vi "ProgressWindowDialog.vi"(0 "LibWriter":refnum<class "LibWriter.lvclass">, 5 "error in (no error)":errorcluster) -> (19 "error out":errorcluster)   [LabVIEW 2014, in "LibWriter.lvclass"]
uses:
  <resource>/Framework/Providers/Open_GDS/ClassProviders/LibProvider_BaseClassInterface/LibWriter_class/ClassWriter_class/LibWriter.lvclass
  <vilib>/picture/picture.llb/imagedata.ctl
  <resource>/Framework/Providers/Open_GDS/ClassProviders/LibProvider_BaseClassInterface/LibWriter_class/ClassWriter_class/LibWriter.lvclass/LibWriter.ctl
panel:
  out "Message":string
  out "Bar":picture
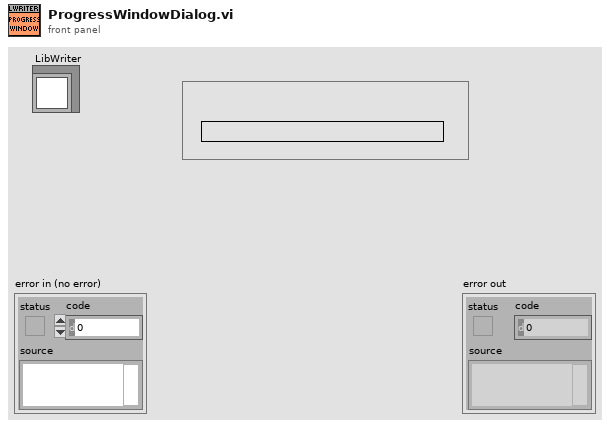
[diagram p1: front panel]
types:
  T1 = typedef "imagedata.ctl" = cluster{"image type":i32, "image depth":i32, "image":u8[], "mask":u8[], "colors":u32[], "Rectangle":cluster{"left":i16, "top":i16, "right":i16, "bottom":i16}}
  T2 = cluster{"i":i32, "end":i32, "Right":bool, "Event":refnum<event-registration>}
  T3 = enum32{"Invalid", "Default", "Floating", "Floating/Auto-Hide", "Modal"}
  T4 = cluster{"left":i16, "top":i16, "right":i16, "bottom":i16}
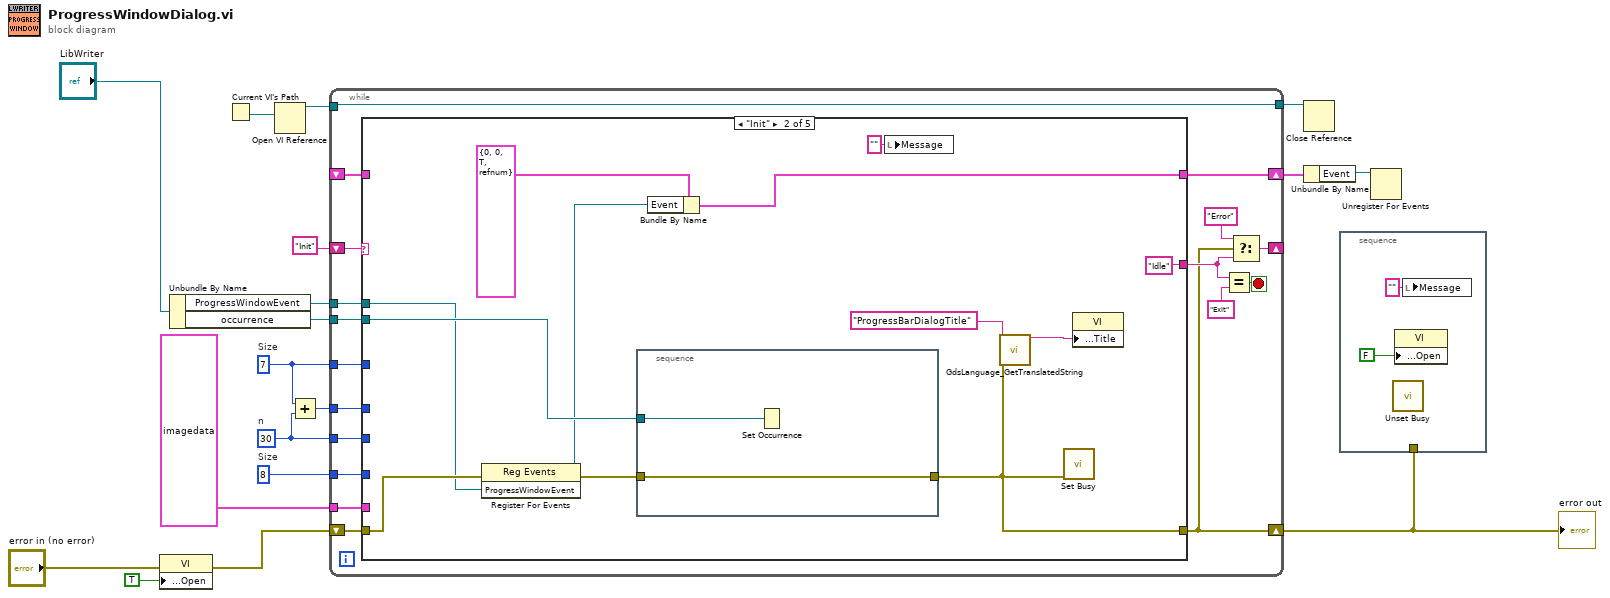
[diagram p0: block diagram]
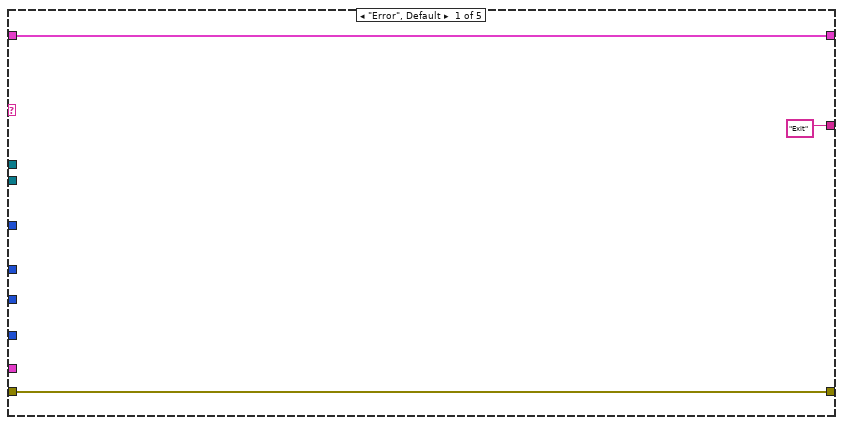
[diagram p2: hidden frame]
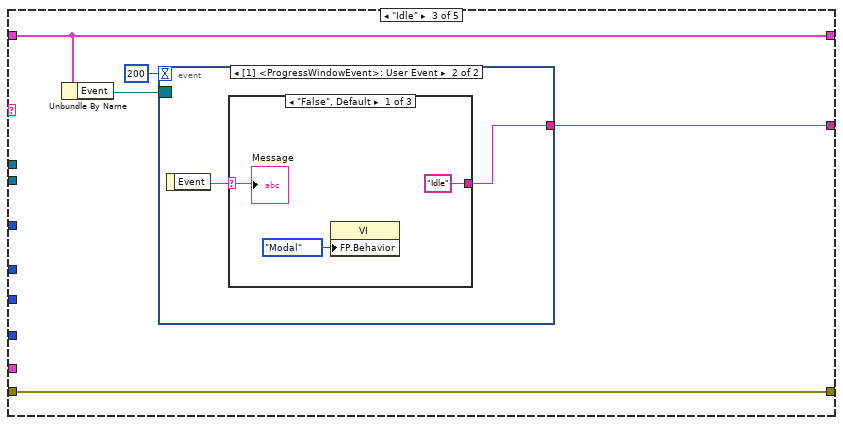
[diagram p3: hidden frame]
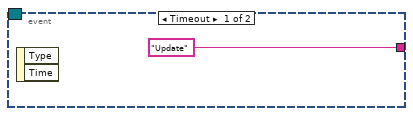
[diagram p4: hidden frame]
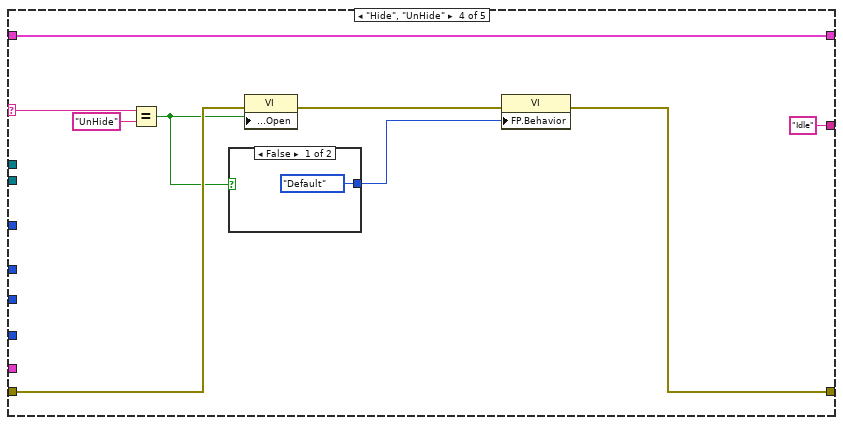
[diagram p7: hidden frame]
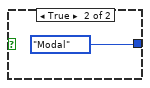
[diagram p8: hidden frame]
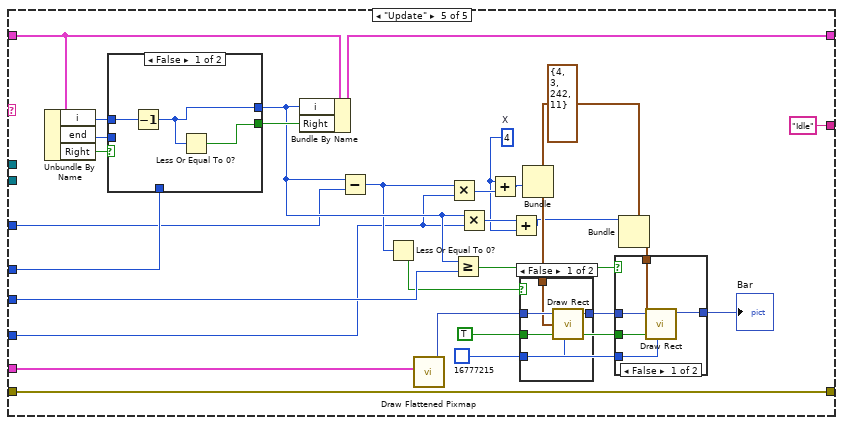
[diagram p9: hidden frame]
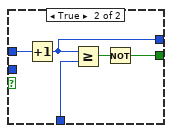
[diagram p12: hidden frame]
diagram:
  w11 = 7  # Size
  w12 = 8  # Size
  w10 = 30  # n
  n1 = property class="VI"(error in="error in (no error)", "Front Panel.Open"=TRUE ("Front Panel Window:Open")) -> (error out=w6:errorcluster)  [unwired: 1 in, 1 out]
  n2 = Unbundle By Name("LibWriter") -> ("ProgressWindowEvent"=w16:refnum<user-event>, "occurrence"=w13:refnum<k4>)
  n3 = Current VI's Path() -> (path=w2:path)
  n4 = Open VI Reference(vi path=w2) -> (vi reference=w3:refnum<vi>)  [unwired: 5 in, 1 out]
  n5 = Add(x=w11, y=w10) -> (x+y=w9:i32)
  n6 = while {
    shift-right: [w29] -> w7
    shift-left: w6 -> [w36]
    shift-right: [w34] -> _
    shift-left: "Init" -> [w35]
    shift-right: [w28] -> w15
    shift-left: _ -> [w27]
    tunnel: w16 -> [w26]
    tunnel: w13 -> [w25]
    tunnel: w12 -> [w24]
    tunnel: w10 -> [w23]
    tunnel: w11 -> [w22]
    tunnel: T1 {"image type"=0, "image depth"=24, "image"=array[9555 elements], "mask"=[], "colors"=[], "Rectangle"={"left"=0, "top"=0, "right"=245, "bottom"=13}} ("image data") -> [w21]
    tunnel: w9 -> [w20]
    tunnel: w3 -> [w19]
    tunnel: [w19] -> w1
    stop <- w33 stop-if-true
    n7 = case shown="\"Init\"" w35 {
      selector: w35 -> [_ _ _ w74 _]
      tunnel: w36 -> [w39 w47 w56 w72 w107]
      tunnel: [w39 w41 w56 w68 w107] -> w29
      tunnel: ["Exit" "Idle" w54 "Idle" ("f") "Idle"] -> w30
      tunnel: [w37 w49 w58 w75 w88] -> w28
      tunnel: w27 -> [w37 _ w58 w75 w91]
      tunnel: w26 -> [_ w45 _ _ _]
      tunnel: w25 -> [_ w46 _ _ _]
      tunnel: w24 -> [_ _ _ _ w81]
      tunnel: w23 -> [_ _ _ _ w90]
      tunnel: w22 -> [_ _ _ _ w86]
      tunnel: w21 -> [_ _ _ _ w102]
      tunnel: w20 -> [_ _ _ _ w93]
      frame "Error", Default {
      }
      frame "Init" {
        n8 = register-events(error in=w47, w45) -> (reference out=w44:refnum<event-registration>, error out=w48:errorcluster)  [unwired: 1 in]
        n9 = stacked-sequence {
          tunnel: w48 -> [w53]
          tunnel: [w53] -> w41
          tunnel: w46 -> [w52]
          frame #0 {
            n10 = Set Occurrence(w52) -> ()
          }
        }
        n11 = Bundle By Name(cluster=T2 {"i"=0, "end"=0, "Right"=TRUE, "Event"=refnum}, "Event"=w44) -> (w49:T2)
        n12 = local write "Message"("" ("Message")) -> ()
        n13 = call <resource>:"GdsLanguage_GetTranslatedString.vi"("StringID(s)"="ProgressBarDialogTitle", "error in (no error)"=w41) -> ("FirstStringOut"=w42:string)  [unwired: 14 in, 3 out]
        n14 = call <vilib>:"Set Busy.vi"("error in (no error)"=w41) -> ()  [unwired: 9 in, 2 out]
        n15 = property class="VI"("Front Panel.Title"=w42) -> ()  [unwired: 2 in, 2 out]
      }
      frame "Idle" {
        n16 = Unbundle By Name(w58) -> ("Event"=w57:refnum<event-registration>)
        n17 = event shown="[1] <ProgressWindowEvent>: User Event" {
          selector: w57 -> [_ _]
          dyn-events: _ -> [_ _]
          timeout: 200 -> [_ _]
          tunnel: ["Update" w60] -> w54
          event Timeout {
            n18 = event-data() -> ()  [unwired: 1 in, 2 out]
          }
          event User Event {
            n19 = event-data() -> ("Event"=w61:string)  [unwired: 1 in]
            n20 = case shown="\"False\", Default" w61 {
              selector: w61 -> [w64 w65 w66]
              tunnel: ["Idle" ("f") w65 w66] -> w60
              frame "False", Default {
                n21 = property class="VI"("FP.Behavior"=T3."Modal" ("Front Panel Window:Behavior")) -> ()  [unwired: 2 in, 2 out]
                "Message" <- w64
              }
              frame "Exit" {
              }
              frame "Hide", "UnHide" {
              }
            }
          }
        }
      }
      frame "Hide", "UnHide" {
        n22 = Equal?(x=w74, y="UnHide") -> (x = y?=w67:bool)
        n23 = case shown="False" w67 {
          tunnel: [T3."Default" ("Front Panel Window:Behavior") T3."Modal" ("Front Panel Window:Behavior")] -> w70
          frame False {
          }
          frame True {
          }
        }
        n24 = property class="VI"(error in=w72, "Front Panel.Open"=w67) -> (error out=w69:errorcluster)  [unwired: 1 in, 1 out]
        n25 = property class="VI"(error in=w69, "FP.Behavior"=w70) -> (error out=w68:errorcluster)  [unwired: 1 in, 1 out]
      }
      frame "Update" {
        w98 = T4 {"left"=4, "top"=3, "right"=242, "bottom"=11} ("rect")
        w79 = 4  # X
        w96 = u32 16777215 ("color(black)")
        w95 = TRUE ("fill?(F)")
        n26 = Unbundle By Name(w91) -> ("i"=w103:i32, "end"=w104:i32, "Right"=w105:bool)
        n27 = case shown="False" w105 {
          tunnel: w104 -> [_ _]
          tunnel: w103 -> [w122 w127]
          tunnel: w93 -> [_ w126]
          tunnel: [w120 w124] -> w92
          tunnel: [w121 w123] -> w87
          frame False {
            n28 = Decrement(x=w122) -> (x-1=w121:i32)
            n29 = Less Or Equal To 0?(x=w121) -> (x <= 0?=w120:bool)
          }
          frame True {
            n30 = Increment(x=w127) -> (x+1=w123:i32)
            n31 = Greater Or Equal?(x=w123, y=w126) -> (x >= y?=w125:bool)
            n32 = Not(x=w125) -> (.not. x?=w124:bool)
          }
        }
        n33 = Bundle By Name(cluster=w91, "i"=w87, "Right"=w92) -> (w88:T2)
        n34 = Subtract(x=w87, y=w86) -> (x-y=w82:i32)
        n35 = Less Or Equal To 0?(x=w82) -> (x <= 0?=w85:bool)
        n36 = call <vilib>:"Draw Flattened Pixmap.vi"("image data"=w102) -> ("new picture"=w101:picture)  [unwired: 8 in]
        n37 = Multiply(x=w82, y=w81) -> (x*y=w80:i32)
        n38 = Greater Or Equal?(x=w87, y=w90) -> (x >= y?=w89:bool)
        n39 = Multiply(x=w87, y=w81) -> (x*y=w84:i32)
        n40 = Add(x=w79, y=w80) -> (x+y=w78:i32)
        n41 = Add(x=w84, y=w79) -> (x+y=w83:i32)
        n42 = Bundle(cluster=w98, "right"=w78) -> (w100:T4)  [unwired: 3 in]
        n43 = case shown="False" w85 {
          tunnel: w101 -> [w112 w113]
          tunnel: w100 -> [w111 _]
          tunnel: [w110 w113] -> w99
          tunnel: w96 -> [w109 _]
          tunnel: w95 -> [w108 _]
          frame False {
            n44 = call <vilib>:"Draw Rect.vi"("picture"=w112, "rect"=w111, "fill?(F)"=w108, "color(black)"=w109) -> ("new picture"=w110:picture)  [unwired: 5 in]
          }
          frame True {
          }
        }
        n45 = Bundle(cluster=w98, "left"=w83) -> (w97:T4)  [unwired: 3 in]
        n46 = case shown="False" w89 {
          tunnel: w99 -> [w118 w119]
          tunnel: w97 -> [w117 _]
          tunnel: w96 -> [w116 _]
          tunnel: w95 -> [w115 _]
          tunnel: [w114 w119] -> w94
          frame False {
            n47 = call <vilib>:"Draw Rect.vi"("picture"=w118, "rect"=w117, "fill?(F)"=w115, "color(black)"=w116) -> ("new picture"=w114:picture)  [unwired: 5 in]
          }
          frame True {
          }
        }
        "Bar" <- w94
      }
    }
    n48 = Equal?(x=w30, y="Exit") -> (x = y?=w33:bool)
    n49 = Select(t="Error", s=w29, f=w30) -> (s? t:f=w34:string)
  }
  "error out" <- w7
  n50 = Close Reference(reference=w1) -> ()  [unwired: 1 in, 1 out]
  n51 = Unbundle By Name(w15) -> ("Event"=w14:refnum<event-registration>)
  n52 = stacked-sequence {
    tunnel: w7 -> [_]
    frame #0 {
      n53 = call <vilib>:"Unset Busy.vi"() -> ()  [unwired: 11 in, 1 out]
      n54 = property class="VI"("Front Panel.Open"=FALSE ("Front Panel Window:Open")) -> ()  [unwired: 2 in, 2 out]
      n55 = local write "Message"("" ("Message")) -> ()
    }
  }
  n56 = Unregister For Events(event registration refnum=w14) -> ()  [unwired: 1 in, 1 out]
